vi "ReturnString_to_ReturnList.vi"(3 "error in (no error)":errorcluster, 4 "return string":string) -> (0 "error out":errorcluster, 1 "return list":T1[](array[typedef]))   [LabVIEW 2016, in "PyLVi.lvlib" / "PyLVi.lvclass"]
uses:
  PyLVi.lvclass
  Controls/ArgumentStructure.ctl
  Controls/DescriptorStructure.ctl
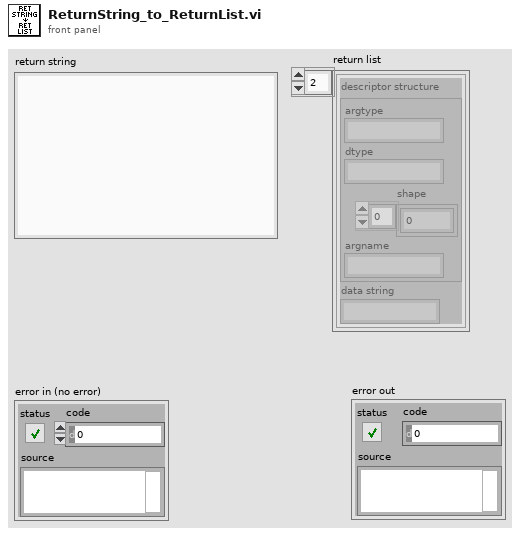
[diagram p1: front panel]
types:
  T1 = typedef "PyLVi.lvlib/PyLVi.lvclass/ArgumentStructure.ctl" = cluster{"descriptor structure":T2, "data string":string}
  T2 = typedef "PyLVi.lvlib/PyLVi.lvclass/DescriptorStructure.ctl" = cluster{"argtype":string, "dtype":string, "shape":u32[], "argname":string}
  T3 = typedef "PyLVi.lvlib/PyLVi.lvclass/ArgumentType.ctl" = enum8{"bool", "numeric", "string", "dict", "ndarray", "ndarray2d"}
  T4 = typedef "PyLVi.lvlib/PyLVi.lvclass/DataType.ctl" = enum16{"bool", "string", "int16", "int32", "float32", "float64", "complex128"}
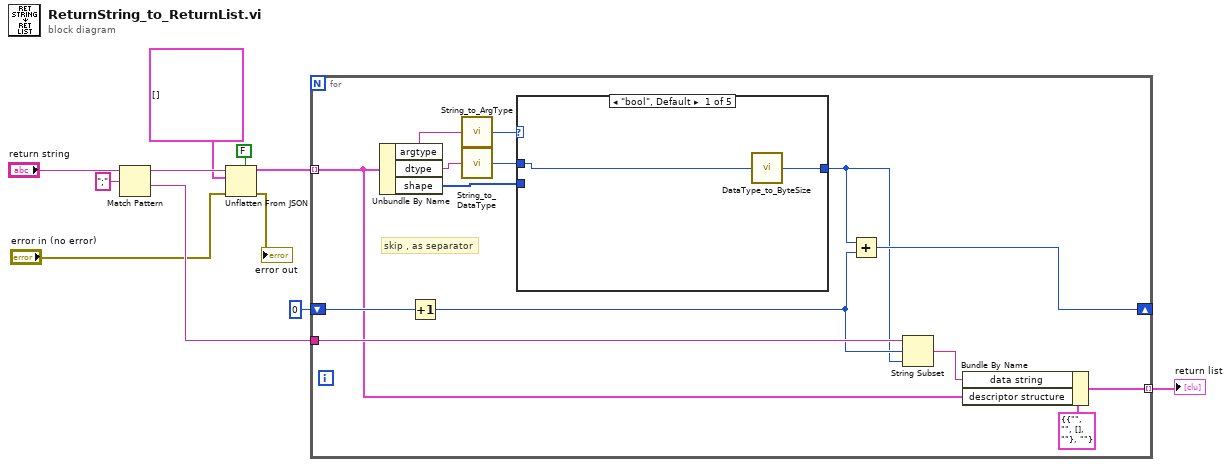
[diagram p0: block diagram]
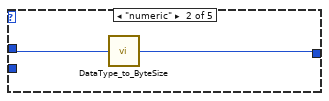
[diagram p2: hidden frame]
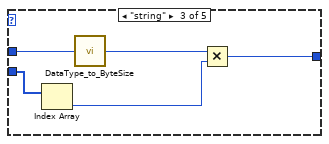
[diagram p3: hidden frame]
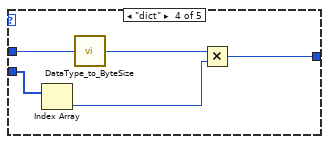
[diagram p4: hidden frame]
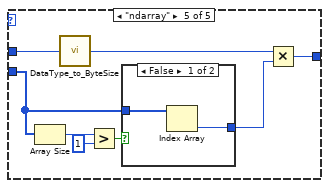
[diagram p5: hidden frame]
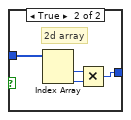
[diagram p6: hidden frame]
diagram:
  n1 = Match Pattern(string="return string", regular expression=";") -> (before substring=w9:string, after substring=w5:string)  [unwired: 1 in, 2 out]
  n2 = Unflatten From JSON(enable LabVIEW extensions? (T)=FALSE, JSON string=w9, type and defaults=T2[] [], error in (no error)="error in (no error)") -> (value=w6:T2[], error out=→"error out":errorcluster)  [unwired: 3 in]
  n3 = for {
    tunnel: w6 -> [w15] mode=indexing
    shift-right: [w18] -> _
    shift-left: u32 0 -> [w19]
    tunnel: w5 -> [w20]
    tunnel: [w14] -> w4 mode=indexing
    # "skip , as separator"
    n4 = Unbundle By Name(w15) -> ("argtype"=w25:string, "dtype"=w23:string, "shape"=w22:u32[])
    n5 = Increment(x=w19) -> (x+1=w13:u32)
    n6 = call "String_to_ArgType.vi"("arg type string"=w25) -> ("arg type"=w24:T3)  [unwired: 4 in]
    n7 = call "String_to_DataType.vi"("data type string"=w23) -> ("data type"=w21:T4)  [unwired: 4 in]
    n8 = case shown="\"bool\", Default" w24 {
      tunnel: w22 -> [_ _ w32 w37 w41]
      tunnel: w21 -> [w26 w29 w34 w39 w47]
      tunnel: [w27 w28 w30 w35 w45] -> w12
      frame "bool", Default {
        n9 = call "DataType_to_ByteSize.vi"("data type"=w26) -> ("byte size"=w27:u32)  [unwired: 4 in]
      }
      frame "numeric" {
        n10 = call "DataType_to_ByteSize.vi"("data type"=w29) -> ("byte size"=w28:u32)  [unwired: 4 in]
      }
      frame "string" {
        n11 = Index Array(array=w32) -> (element=w31:u32)  [unwired: 1 in]
        n12 = call "DataType_to_ByteSize.vi"("data type"=w34) -> ("byte size"=w33:u32)  [unwired: 4 in]
        n13 = Multiply(x=w33, y=w31) -> (x*y=w30:u32)
      }
      frame "dict" {
        n14 = Index Array(array=w37) -> (element=w36:u32)  [unwired: 1 in]
        n15 = call "DataType_to_ByteSize.vi"("data type"=w39) -> ("byte size"=w38:u32)  [unwired: 4 in]
        n16 = Multiply(x=w38, y=w36) -> (x*y=w35:u32)
      }
      frame "ndarray" {
        n17 = Array Size(array=w41) -> (size(s)=w44:i32)
        n18 = call "DataType_to_ByteSize.vi"("data type"=w47) -> ("byte size"=w46:u32)  [unwired: 4 in]
        n19 = Greater?(x=w44, y=1) -> (0:w42:bool)
        n20 = case shown="False" w42 {
          tunnel: w41 -> [w49 w53]
          tunnel: [w48 w50] -> w40
          frame False {
            n21 = Index Array(array=w49) -> (element=w48:u32)  [unwired: 1 in]
          }
          frame True {
            # "2d array"
            n22 = Index Array(array=w53) -> (element #1=w52:u32, element #2=w51:u32)  [unwired: 2 in]
            n23 = Multiply(x=w52, y=w51) -> (x*y=w50:u32)
          }
        }
        n24 = Multiply(x=w46, y=w40) -> (x*y=w45:u32)
      }
    }
    n25 = Add(x=w12, y=w13) -> (x+y=w18:u32)
    n26 = String Subset(string=w20, offset (0)=w13, length (rest)=w12) -> (substring=w16:string)
    n27 = Bundle By Name(cluster=T1 {"descriptor structure"={"argtype"="", "dtype"="", "shape"=[], "argname"=""}, "data string"=""} ("argument structure"), "data string"=w16, "descriptor structure"=w15) -> (w14:T1)
  }
  "return list" <- w4
